vi "Try 1.vi"() -> ()   [LabVIEW 2018]
panel:
  in  "Freq Min":dbl
  in  "Freq Max":dbl
  out "Waveform Chart":dynamicdata(graph)
  in  "Read Voltage Min":dbl
  in  "Read Voltage Max":dbl
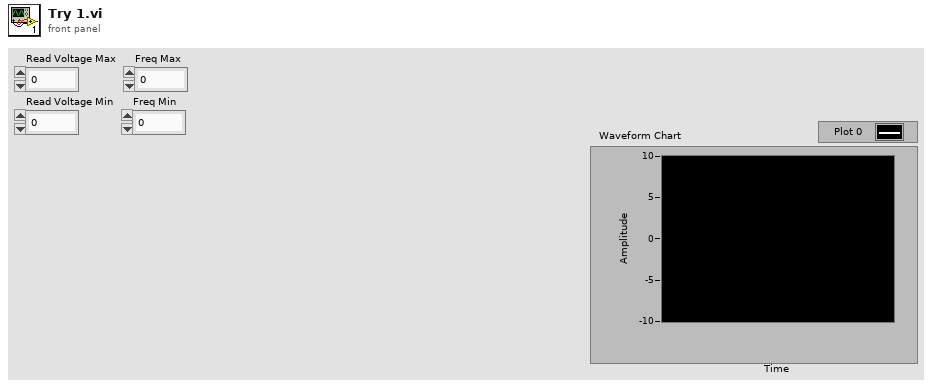
[diagram p1: front panel]
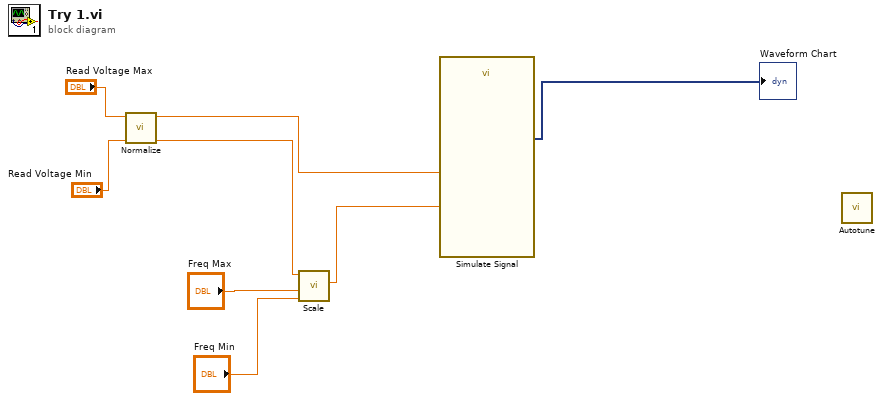
[diagram p0: block diagram]
diagram:
  n1 = call "Normalize.vi"("Min"="Read Voltage Min", "Max"="Read Voltage Max") -> ("A1"=w6:dbl, "A0"=w3:dbl)  [unwired: 8 in]
  n2 = call "Scale.vi"("Min"="Freq Min", "Max"="Freq Max", "Normalized Input"=w6) -> ("Scaled Output"=w5:dbl)  [unwired: 8 in]
  n3 = call "Simulate Signal"("Frequency"=w5, "Amplitude"=w3) -> ("Sine"=→"Waveform Chart":dynamicdata)  [unwired: 12 in, 1 out]
  n4 = call "Autotune.vi"() -> ()  [unwired: 10 in, 2 out]
